vi "HI.vi"   [LabVIEW 2012]
uses:
  Conveyer Belt/Conveyer Belt Global Data.vi
  Drive/Drive Global Data.vi
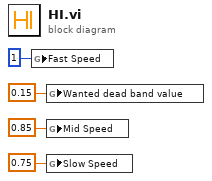
[diagram p0: block diagram]
diagram:
  n1 = global write "Conveyer Belt Global Data.vi" "Fast Speed"(1) -> ()
  n2 = global write "Drive Global Data.vi" "Wanted dead band value"(0.15) -> ()
  n3 = global write "Conveyer Belt Global Data.vi" "Mid Speed"(0.85) -> ()
  n4 = global write "Conveyer Belt Global Data.vi" "Slow Speed"(0.75) -> ()
